vi "_Register Group.vi"(8 "error in (no error)":errorcluster, 10 "Group":refnum<class "Group.lvclass">, 11 "Loop Data In":T1) -> (0 "error out":errorcluster, 3 "Loop Data":T1)   [LabVIEW 2020, in "Vecto.lvlib" / "RemoteDataService.lvclass"]
uses:
  RemoteDataService.lvclass
  Loop Data.ctl
  SequenceCountService/SequenceCountService.lvclass
  Published Group.ctl
  Packet.ctl
  <vilib>/IlluminatedG/IG Protoc/LV-Proto/Message/Message.lvclass
  Group/Group.lvclass
  Group Config/Group Config.lvclass
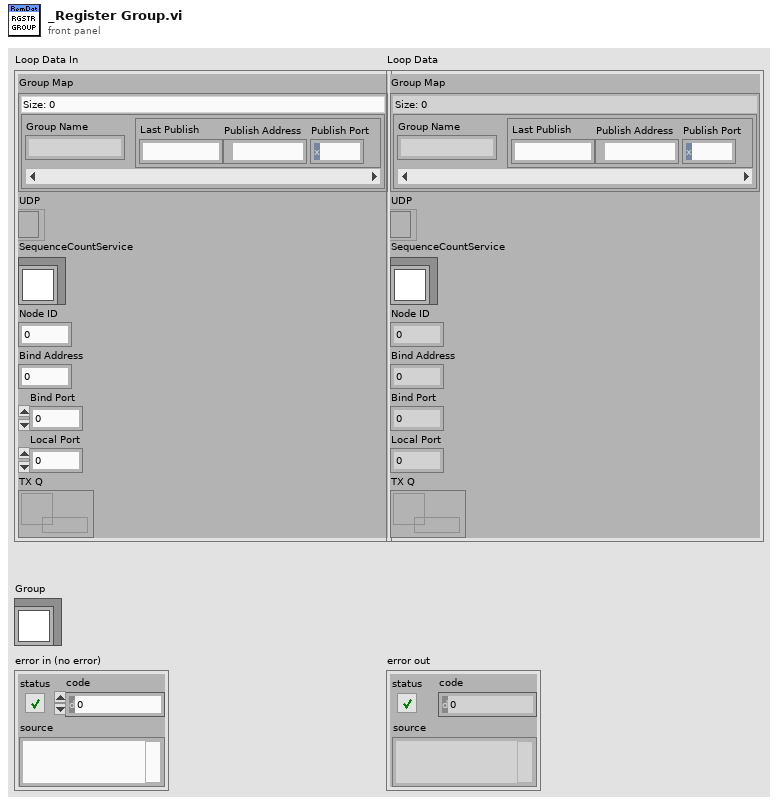
[diagram p1: front panel]
types:
  T1 = typedef "Vecto.lvlib/RemoteDataService.lvclass/Loop Data.ctl" = cluster{"Group Map":map{string, T2}, "UDP":refnum<k16>, "SequenceCountService":refnum<class "SequenceCountService.lvclass">, "Node ID":u32, "Bind Address":u32, "Bind Port":u16, "Local Port":u16, "TX Q":refnum<queue>}
  T2 = typedef "Vecto.lvlib/RemoteDataService.lvclass/Published Group.ctl" = cluster{"Last Publish":dbl, "Publish Address":u32, "Publish Port":u16}
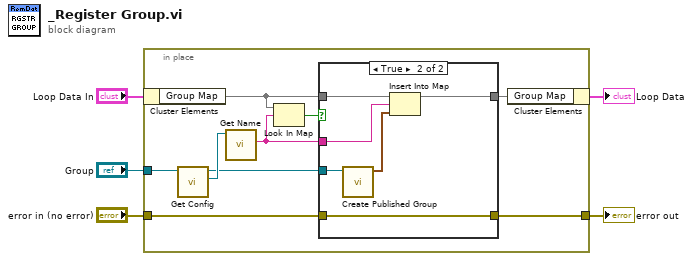
[diagram p0: block diagram]
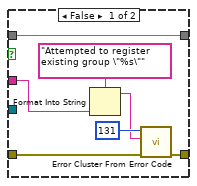
[diagram p2: hidden frame]
diagram:
  n1 = in-place {
    in-place-border: "Group" -> [w14]
    in-place-border: "error in (no error)" -> [w8]
    in-place-border: [w6] -> w1
    n2 = in-place-cluster #1("Loop Data In") -> ("Group Map"=w11:map{string, T2})
    n3 = call "Get Config.vi"("Group in"=w14) -> ("Config"=w13:refnum<class "Group Config.lvclass">, "Group out"=w10:refnum<class "Group.lvclass">)  [unwired: 8 in, 1 out]
    n4 = call "Get Name.vi"("Group Config in"=w13) -> ("Name"=w9:string)  [unwired: 8 in, 2 out]
    n5 = Look In Map(map=w11, key=w9) -> (key not found?=w12:bool)  [unwired: 1 in, 1 out]
    n6 = case shown="True" w12 {
      tunnel: w11 -> [w21 w25]
      tunnel: w10 -> [_ w23]
      tunnel: w9 -> [w18 w26]
      tunnel: w8 -> [w20 w27]
      tunnel: [w21 w24] -> w7
      tunnel: [w15 w27] -> w6
      frame False {
        n7 = Format Into String(format string="Attempted to register existing group \"%s\"", w18) -> (resulting string=w16:string)  [unwired: 2 in, 1 out]
        n8 = call <vilib>:"Error Cluster From Error Code.vi"("error in (no error)"=w20, "error message (\"\")"=w16, "error code (0)"=131) -> ("error out"=w15:errorcluster)  [unwired: 6 in]
      }
      frame True {
        n9 = call "Create Published Group.vi"("Group"=w23) -> ("Published Group"=w22:T2)  [unwired: 10 in]
        n10 = Insert Into Map(map in=w25, key=w26, value=w22) -> (map out=w24:map{string, T2})  [unwired: 2 out]
      }
    }
    n11 = in-place-cluster #1("Group Map"=w7) -> (→"Loop Data":T1)
  }
  "error out" <- w1
